vi "Dax_RadValsBP2_2.vi"(11 "Daxsonics":refnum<visa-resource-name>) -> (1 "Freq (MHz)":u16(ring)=5 items=["10", "12", "14", "16", "18", "20", "25", "30", "35", "40", "45"], 2 "Amp (V)":u16(ring) items=["0", "10", "20", "30", "40", "50", "60", "70", "80", "90", "100", "110", "120", "130", "140", "150", "160", "170", "180", "190"], 3 "Gains":u16[](array[ring]) items=["22", "25", "28", "31", "34", "37", "40", "43", "46", "49", "52", "55", "58", "61", "64"])   [LabVIEW 2022 SP3]
uses:
  ScanningControl/Pulsers/PulserGlobals.vi
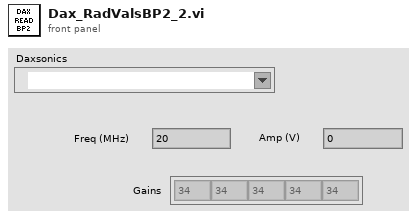
[diagram p1: front panel]
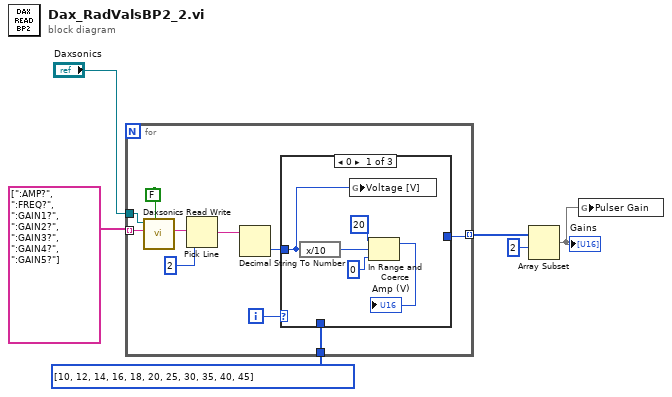
[diagram p0: block diagram]
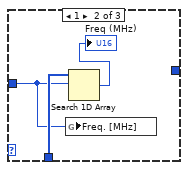
[diagram p2: hidden frame]
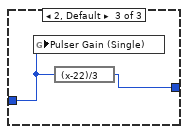
[diagram p3: hidden frame]
diagram:
  n1 = for {
    tunnel: string[] [":AMP?", ":FREQ?", ":GAIN1?", ":GAIN2?", ":GAIN3?", ":GAIN4?", ":GAIN5?"] -> [w13] mode=indexing
    tunnel: i32[] [10, 12, 14, 16, 18, 20, 25, 30, 35, 40, 45] -> [w14]
    tunnel: "Daxsonics" -> [w9]
    tunnel: [w7] -> w4 mode=indexing
    i -> [w16]
    n2 = call "Daxsonics Read Write.vi"("Daxsonics Name"=FALSE ("Enable Termination\nChar (T)"), "write buffer"=w13, "VISA resource name"=w9) -> ("read buffer"=w12:string)  [unwired: 6 in, 2 out]
    n3 = Pick Line(multi-line string=w12, line index=2) -> (output string=w11:string)  [unwired: 1 in]
    n4 = Decimal String To Number(string=w11) -> (number=w15:i32)  [unwired: 2 in, 1 out]
    n5 = case shown="0" w16 {
      tunnel: w15 -> [w18 w23 w26]
      tunnel: w14 -> [_ w24 _]
      tunnel: [_ _ w25] -> w7
      frame 0 {
        n6 = expression code="x/10"(w18) -> (w21:i32)
        n7 = global write "PulserGlobals.vi" "Voltage [V]"(w18) -> ()
        n8 = In Range and Coerce(upper limit=20, x=w21, lower limit=0) -> (coerced(x)=→"Amp (V)":i32)  [unwired: 1 out]
      }
      frame 1 {
        n9 = global write "PulserGlobals.vi" "Freq. [MHz]"(w23) -> ()
        n10 = Search 1D Array(1D array=w24, element=w23) -> (index of element=→"Freq (MHz)":i32)  [unwired: 1 in]
      }
      frame 2, Default {
        n11 = global write "PulserGlobals.vi" "Pulser Gain (Single)"(w26) -> ()
        n12 = expression code="(x-22)/3"(w26) -> (w25:i32)
      }
    }
  }
  n13 = Array Subset(array=w4, index=2) -> (w1:i32[])  [unwired: 1 in]
  "Gains" <- w1
  n14 = global write "PulserGlobals.vi" "Pulser Gain"(w1) -> ()
